vi "InsightDisplay.vi"(10 "Zone 2 Data":string[](array[string]), 11 "Zone 1 Data":string[](array[string])) -> ()   [LabVIEW 2013]
uses:
  <vilib>/Rock Robotics/SystemInterfaces/Typedef/FPGA_TypedefDigitalModule.ctl
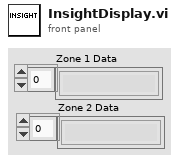
[diagram p1: front panel]
types:
  T1 = enum16{"FOUR_ZONES", "ONE_ZONE_TWO_LINES", "TWO_ZONES_ONE_LINE"}
  T2 = typedef "FPGA_TypedefDigitalModule.ctl" = enum16{"Digital Module 1", "Digital Module 2"}
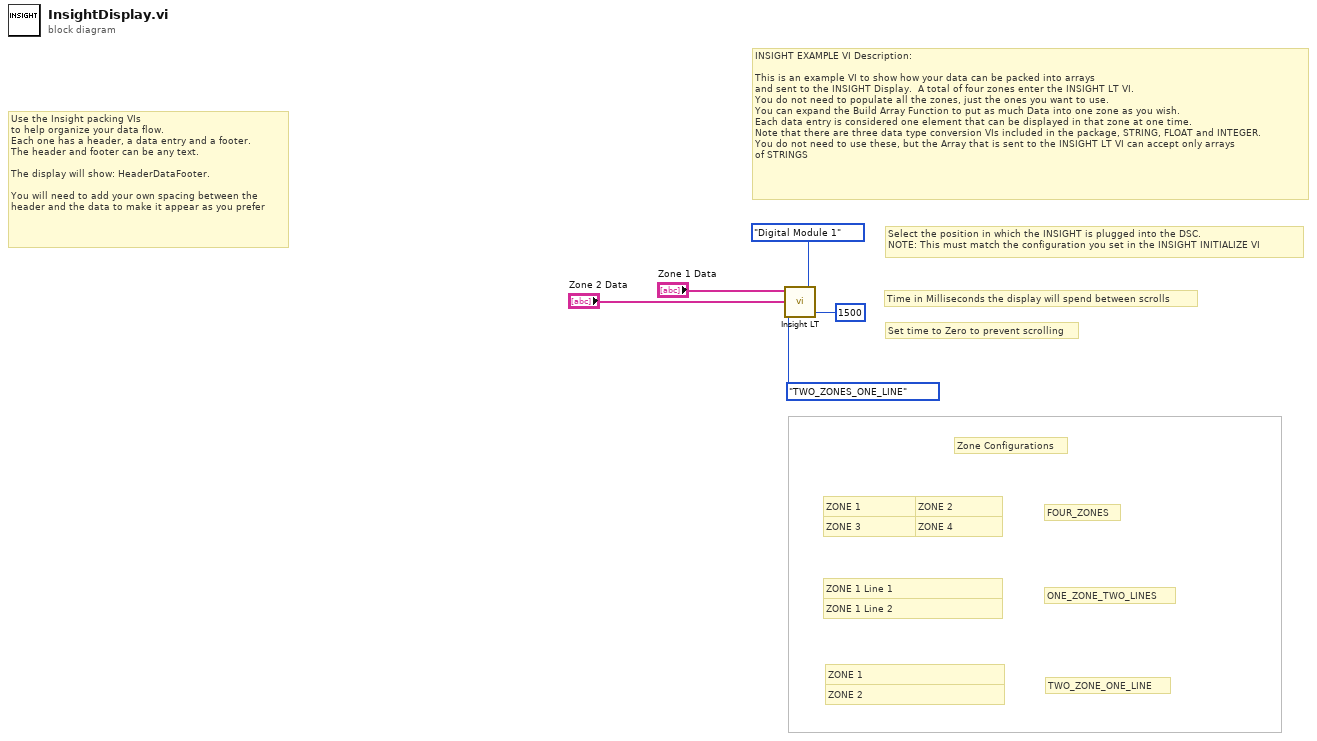
[diagram p0: block diagram]
diagram:
  # "Set time to Zero to prevent scrolling"
  # "Use the Insight packing VIs\nto help organize your data flow.\nEach one has a header, a data entry and a footer.\nThe header and footer can be any text.\n\nThe display will show: HeaderDataFooter.\n\nYou will need to add your own spacing between the \nheader and the data to make it appear as you prefer"
  # "TWO_ZONE_ONE_LINE"
  # "ONE_ZONE_TWO_LINES"
  # "FOUR_ZONES"
  # "Zone Configurations"
  # "ZONE 4"
  # "ZONE 2"
  # "ZONE 3"
  # "ZONE 1"
  # "ZONE 1 Line 2"
  # "ZONE 1 Line 1"
  # "ZONE 2"
  # "ZONE 1"
  # "Time in Milliseconds the display will spend between scrolls"
  # "Select the position in which the INSIGHT is plugged into the DSC.\nNOTE: This must match the configuration you set in the INSIGHT INITIALIZE VI"
  # "INSIGHT EXAMPLE VI Description:\n\nThis is an example VI to show how your data can be packed into arrays\nand sent to the INSIGHT Display.  A total of four zones enter the INSIGHT LT VI. \nYou do not need to populate all the zones, just the ones you want to use.\nYou can expand the Build Array Function to put as much Data into one zone as you wish.\nEach data entry is considered one element that can be displayed in that zone at one time.\nNote that there are three data type conversion VIs included in the package, STRING, FLOAT and INTEGER.\nYou do not need to use these, but the Array that is sent to the INSIGHT LT VI can accept only arrays\nof STRINGS"
  n1 = call "Insight LT.vi"("Scroll Timing"=1500, "ZONE \nCONFIGURATION"=T1."TWO_ZONES_ONE_LINE" ("ZONE \nCONFIGURATION"), "Digital Module"=FPGA_TypedefDigitalModule."Digital Module 1", "Zone 2 Data"="Zone 2 Data", "Zone 1 Data"="Zone 1 Data") -> ()  [unwired: 2 in]
